vi "Send Data for UI.vi"(0 "Measure Call Context in":refnum<class "Measure Call Context.lvclass">, 1 "fpga interface in":refnum<k20>, 2 "Embedded Data":T2, 3 "Last displayed image data":u32[](array[numeric]), 5 "FrameCount":u64, 7 "registers":string[][](array[string])=[["0x10", "0x2030", "0x01f0"], ["0x10", "0x3120", "0x0802"]], 9 "References":T4, 11 "error in":errorcluster, 12 "Status data":T6, 13 "SOURCE RATE (fps)":dbl, 14 "Active Channel":string) -> (4 "output cluster":T1={"ACQ. IN PROGRESS"=FALSE, "IMAGE PIXEL DATA"=[], "ACQ. DURATION (s)"=0.0, "SOURCE RATE (fps)"=0.0, "BYTES ACQUIRED"=0, "FRAME COUNT"=0, "POC VOLTAGE (V)"=0.0, "POC CURRENT (A)"=0.0, "ERROR"=FALSE, "STATE MESSAGE"="Initializing...", "IMAGE DATA"="", "OOB gRPC Port"=0, "HEIGHT"=0, "WIDTH"=0, "FRAME COUNT BYTES"=[], "REGISTERS"=[], "COUNT LENGTH"=0} {"BYTES ACQUIRED" format="%#.6p"}, 15 "error out":errorcluster)   [LabVIEW 2025, in "Automotive Vision.lvclass"]
doc: "Handles data transfer to the UI."
uses:
  Automotive Vision.lvclass
  <vilib>/Plug-In SDKs/Measurements/Measure Call Context/Measure Call Context.lvclass
  <instrlib>/FlexRIO/CSI-2/v2/Common/Types/LLP Data Type.ctl
  embedded data.ctl
  embedded data item.ctl
  Measurement Results.ctl
  Automotive Vision.lvclass/Automotive Vision.ctl
  <instrlib>/FlexRIO/CSI-2/v2/Common/NI CSI-2 API Common v2.lvlib
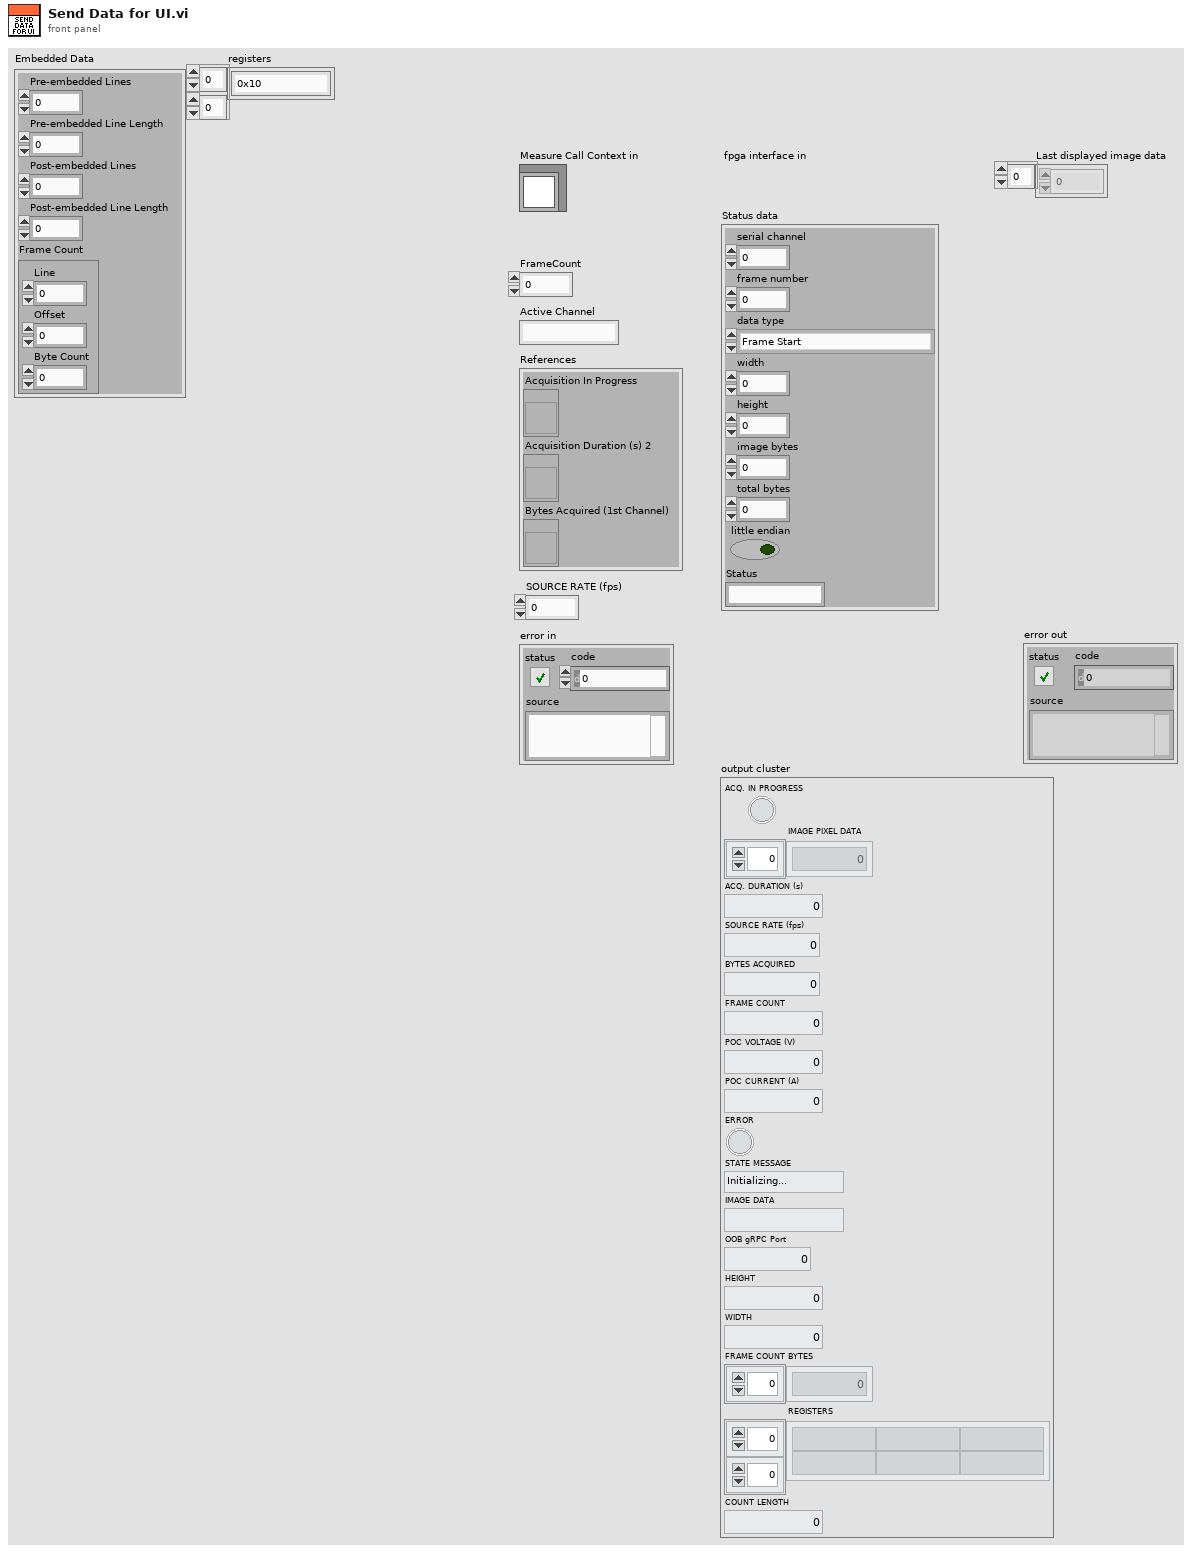
[diagram p1: front panel]
types:
  T1 = typedef "Automotive Vision.lvclass/Measurement Results.ctl" = cluster{"ACQ. IN PROGRESS":bool, "IMAGE PIXEL DATA":u32[], "ACQ. DURATION (s)":dbl, "SOURCE RATE (fps)":dbl, "BYTES ACQUIRED":u64, "FRAME COUNT":u64, "POC VOLTAGE (V)":dbl, "POC CURRENT (A)":dbl, "ERROR":bool, "STATE MESSAGE":string, "IMAGE DATA":string, "OOB gRPC Port":i32, "HEIGHT":u64, "WIDTH":u64, "FRAME COUNT BYTES":u32[], "REGISTERS":string[][], "COUNT LENGTH":u64}
  T2 = typedef "Automotive Vision.lvclass/embedded data.ctl" = cluster{"Pre-embedded Lines":dbl, "Pre-embedded Line Length":dbl, "Post-embedded Lines":dbl, "Post-embedded Line Length":dbl, "Frame Count":T3}
  T3 = typedef "Automotive Vision.lvclass/embedded data item.ctl" = cluster{"Line":dbl, "Offset":dbl, "Byte Count":dbl}
  T4 = cluster{"Acquisition In Progress":refnum<vi>, "Acquisition Duration (s) 2":refnum<vi>, "Bytes Acquired (1st Channel)":refnum<vi>}
  T5 = typedef "NI CSI-2 API Common v2.lvlib/LLP Data Type.ctl" = enum8{"Frame Start", "Frame End", "Line Start", "Line End", "End of Transmission", "Reserved 0", "Reserved 1", "Reserved 2", "Generic Short Packet 1", "Generic Short Packet 2", "Generic Short Packet 3", "Generic Short Packet 4", "Generic Short Packet 5", "Generic Short Packet 6", "Generic Short Packet 7", "Generic Short Packet 8", "Null", "Blanking Data", "Embedded 8-bit non Image Data", "Generic Long Packet 1", "Generic Long Packet 2", "Generic Long Packet 3", "Generic Long Packet 4", "Reserved 3", "YUV420 8-bit", "YUV420 10-bit", "Legacy YUV420 8-bit", "Reserved 4", "YUV420 8-bit Chroma Shifted", "YUV420 10-bit Chroma Shifted", "YUV422 8-bit", "YUV422 10-bit", "RGB444", "RGB555", "RGB565", "RGB666", "RGB888", "Reserved 5", "Reserved 6", "RAW 24", "RAW 6", "RAW 7", "RAW 8", "RAW 10", "RAW 12", "RAW 14", "RAW 16", "RAW 20", "User Defined 8-bit Data 1", "User Defined 8-bit Data 2", "User Defined 8-bit Data 3", "User Defined 8-bit Data 4", "User Defined 8-bit Data 5", "User Defined 8-bit Data 6", "User Defined 8-bit Data 7", "User Defined 8-bit Data 8", "USL Command", "Reserved 7", "Reserved 8", "Reserved 9", "Reserved 10", "Reserved 11", "Reserved 12", "LRTE EPD Spacer"}
  T6 = cluster{"serial channel":fxp<+,3,3>, "frame number":u16, "data type":T5, "width":u16, "height":u16, "image bytes":u32, "total bytes":u32, "little endian":bool, "Status":string}
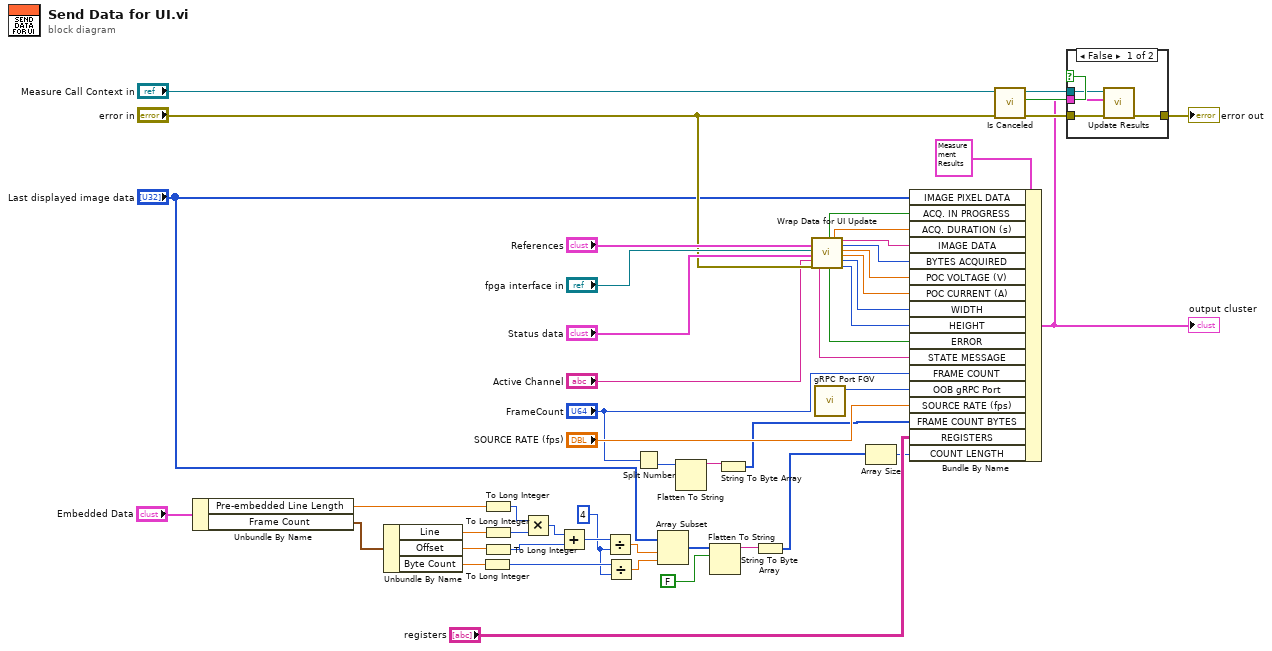
[diagram p0: block diagram]
diagram:
  w10 = 4 ("y")
  n1 = Unbundle By Name("Embedded Data") -> ("Pre-embedded Line Length"=w21:dbl, "Frame Count"=w25:T3)
  n2 = Unbundle By Name(w25) -> ("Line"=w19:dbl, "Offset"=w17:dbl, "Byte Count"=w15:dbl)
  n3 = To Long Integer(number=w15) -> (32bit integer=w11:i32)
  n4 = To Long Integer(number=w21) -> (32bit integer=w20:i32)
  n5 = To Long Integer(number=w19) -> (32bit integer=w18:i32)
  n6 = To Long Integer(number=w17) -> (32bit integer=w16:i32)
  n7 = Multiply(x=w20, y=w18) -> (x*y=w24:i32)
  n8 = Add(x=w24, y=w16) -> (x+y=w14:i32)
  n9 = Divide(x=w14, y=w10) -> (x/y=w13:dbl)
  n10 = Divide(x=w11, y=w10) -> (x/y=w12:dbl)
  n11 = Split Number(x="FrameCount") -> (lo(x)=w1:u32)  [unwired: 1 out]
  n12 = Array Subset(array="Last displayed image data", index=w13, length=w12) -> (w7:u32[])
  n13 = Flatten To String(anything=w1) -> (data string=w4:string)  [unwired: 3 in, 2 out]
  n14 = Flatten To String(anything=w7, prepend array or string size? (T)=FALSE) -> (data string=w8:string)  [unwired: 2 in, 2 out]
  n15 = String To Byte Array(string=w4) -> (unsigned byte array=w3:u8[])
  n16 = String To Byte Array(string=w8) -> (unsigned byte array=w5:u8[])
  n17 = call "Wrap Data for UI Update.vi"("References"="References", "fpga inteface in"="fpga interface in", "image metadata"="Status data", "Active Channel"="Active Channel", "error in"="error in") -> ("State message"=w40:string, "Acqusition In Progress"=w35:bool, "status"=w39:bool, "Acquisition Duration"=w36:dbl, "Image Data"=w30:string, "Bytes Acquired"=w31:u64, "PowerOverCoaxCurrent"=w37:dbl, "PowerOverCoaxVoltage"=w38:dbl, "width"=w48:u64, "height"=w49:u64)  [unwired: 5 in]
  n18 = call "gRPC Port FGV.vi"() -> ("Listening Port out"=w47:i32)  [unwired: 11 in]
  n19 = Array Size(array=w5) -> (size(s)=w22:i32)
  n20 = Bundle By Name(cluster=T1 {"ACQ. IN PROGRESS"=FALSE, "IMAGE PIXEL DATA"=[], "ACQ. DURATION (s)"=0.0, "SOURCE RATE (fps)"=0.0, "BYTES ACQUIRED"=0, "FRAME COUNT"=0, "POC VOLTAGE (V)"=0.0, "POC CURRENT (A)"=0.0, "ERROR"=FALSE, "STATE MESSAGE"="", "IMAGE DATA"="", "OOB gRPC Port"=0, "HEIGHT"=0, "WIDTH"=0, "FRAME COUNT BYTES"=[], "REGISTERS"=[], "COUNT LENGTH"=0} ("Measurement Results"), "IMAGE PIXEL DATA"="Last displayed image data", "ACQ. IN PROGRESS"=w35, "ACQ. DURATION (s)"=w36, "IMAGE DATA"=w30, "BYTES ACQUIRED"=w31, "POC VOLTAGE (V)"=w37, "POC CURRENT (A)"=w38, "WIDTH"=w48, "HEIGHT"=w49, "ERROR"=w39, "STATE MESSAGE"=w40, "FRAME COUNT"="FrameCount", "OOB gRPC Port"=w47, "SOURCE RATE (fps)"="SOURCE RATE (fps)", "FRAME COUNT BYTES"=w3, "REGISTERS"="registers", "COUNT LENGTH"=w22) -> (w33:T1)
  "output cluster" <- w33
  n21 = call <vilib>:"Is Canceled.vi"("error in"="error in", "measure call context in"="Measure Call Context in") -> ("error out"=w46:errorcluster, "is canceled?"=w45:bool, "measure call context out"=w44:refnum<class "Measure Call Context.lvclass">)  [unwired: 7 in]
  n22 = case shown="False" w45 {
    tunnel: w33 -> [w54 _]
    tunnel: [w53 w55] -> w34
    tunnel: w44 -> [w52 _]
    tunnel: w46 -> [w51 w55]
    frame False {
      n23 = call <vilib>:"Update Results.vi"("error in"=w51, "measurement results"=w54, "measure call context in"=w52) -> ("error out"=w53:errorcluster)  [unwired: 7 in, 1 out]
    }
    frame True {
    }
  }
  "error out" <- w34
